vi "visa_status.vi"(8 "error in (no error)":errorcluster) -> ()   [LabVIEW 2016]
uses:
  <vilib>/Utility/error.llb/DialogType.ctl
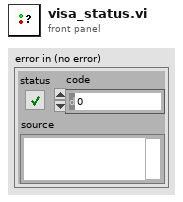
[diagram p1: front panel]
types:
  T1 = typedef "DialogType.ctl" = u16
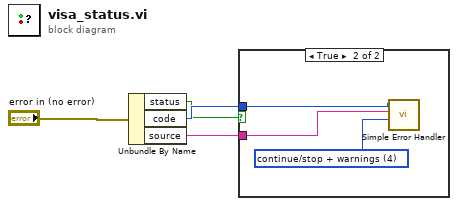
[diagram p0: block diagram]
diagram:
  n1 = Unbundle By Name("error in (no error)") -> ("status"=w3:bool, "code"=w4:i32, "source"=w1:string)
  n2 = case shown="True" w3 {
    tunnel: w4 -> [_ w7]
    tunnel: w1 -> [_ w5]
    frame False {
    }
    frame True {
      w6 = T1 4 items=["no dialog", "OK message", "continue or stop message", "OK message + warnings", "continue/stop + warnings"] ("type of dialog (OK msg:1)")
      n3 = call <vilib>:"Simple Error Handler.vi"("error code (no error:0)"=w7, "error source (\" \")"=w5, "type of dialog (OK msg:1)"=w6) -> ()  [unwired: 2 in, 5 out]
    }
  }
